vi "Import State.vi"(0 "SystemLink connection in":T1, 5 "state filepath":path, 7 "state name":string, 9 "state description":string, 11 "error in (no error)":errorcluster) -> (4 "SystemLink connection out":T1, 6 "state metadata":string, 15 "error out":errorcluster)   [LabVIEW 2017, in "SystemLink_States_API.lvlib"]
doc: "Imports the specified state file (.sls) on disk into the SystemLink server"
uses:
  SystemLink_States_API.lvlib
  _support/systemlink connection.ctl
  <vilib>/httpClient/ClientHandle.ctl
  <vilib>/httpClient/POSTBuffer.vi
  <vilib>/httpClient/LabVIEWHTTPClient.lvlib
panel:
  out "body":string
  out "headers":string
  # "The Import State VI does not work yet.  Need to better research how to implement the Import State HTTP API in LabVIEW\nImport State HTTP API: http://demo.systemlink.io/niapis/?urls.primaryName=Systems%20State%20Manager%20Service#/states/ImportState"
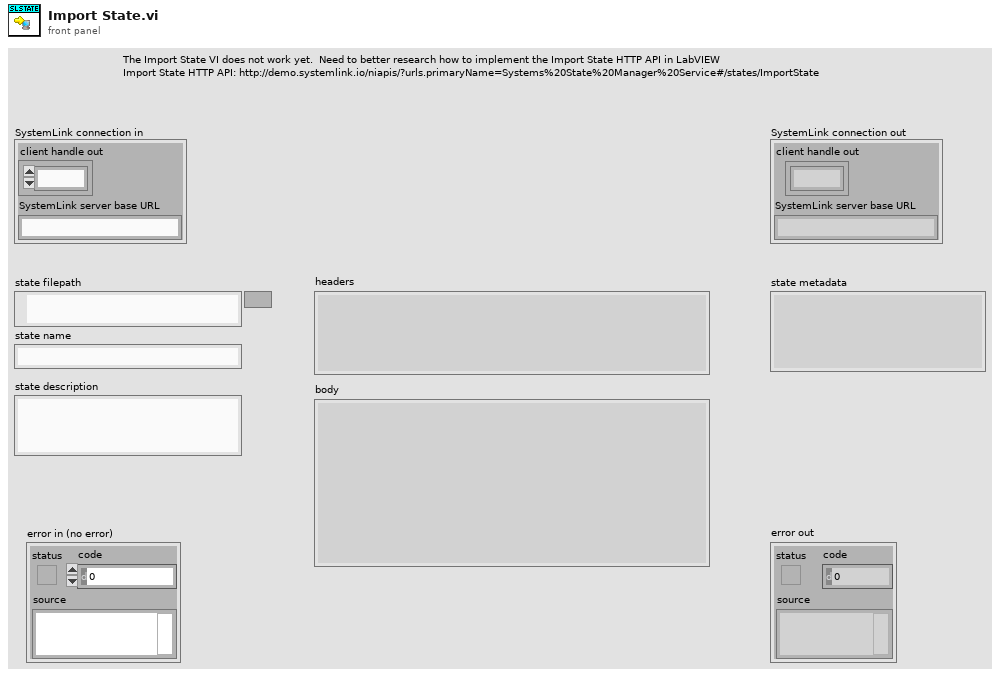
[diagram p1: front panel]
types:
  T1 = typedef "SystemLink_States_API.lvlib/systemlink connection.ctl" = cluster{"client handle out":T2, "SystemLink server base URL":string}
  T2 = typedef "LabVIEWHTTPClient.lvlib/ClientHandle.ctl" = refnum<k1>
  T3 = cluster{"file":string, "name":string, "description":string, "architecture":string}
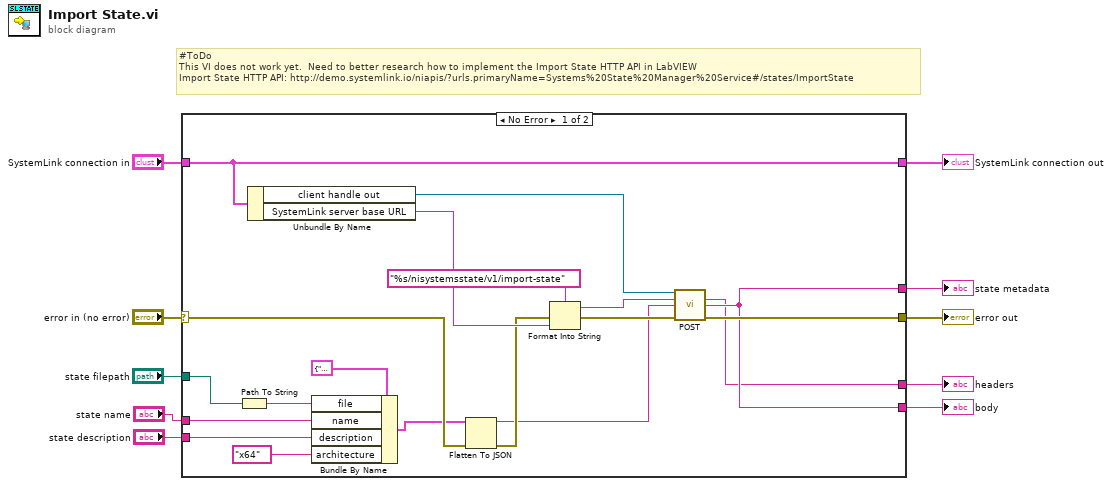
[diagram p0: block diagram]
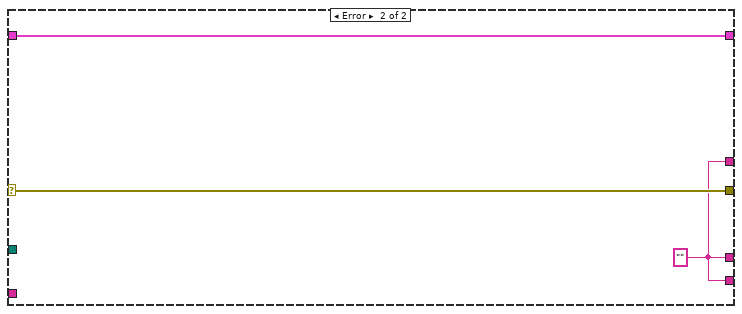
[diagram p2: hidden frame]
diagram:
  # "#ToDo\nThis VI does not work yet.  Need to better research how to implement the Import State HTTP API in LabVIEW\nImport State HTTP API: http://demo.systemlink.io/niapis/?urls.primaryName=Systems%20State%20Manager%20Service#/states/ImportState"
  n1 = case shown="No Error" "error in (no error)" {
    selector: "error in (no error)" -> [w19 w32]
    tunnel: "SystemLink connection in" -> [w21 w30]
    tunnel: [w25 w32] -> w9
    tunnel: [w23 w31] -> w5
    tunnel: [w23 w31] -> w8
    tunnel: [w22 w31] -> w7
    tunnel: "state filepath" -> [w16 _]
    tunnel: [w21 w30] -> w3
    tunnel: "state name" -> [w15 _]
    tunnel: "state description" -> [w13 _]
    frame No Error {
      n2 = Path To String(path=w16) -> (string=w11:string)
      n3 = Unbundle By Name(w21) -> ("client handle out"=w27:T2, "SystemLink server base URL"=w24:string)
      n4 = Bundle By Name(cluster=T3 {"file"="", "name"="", "description"="", "architecture"=""}, "file"=w11, "name"=w15, "description"=w13, "architecture"="x64" ("Combo Box")) -> (w12:T3)
      n5 = Flatten To JSON(anything=w12, error in (no error)=w19) -> (JSON string=w17:string, 11:w18:errorcluster)  [unwired: 1 in]
      n6 = Format Into String(format string="%s/nisystemsstate/v1/import-state", error in=w18, w24) -> (resulting string=w28:string, error out=w26:errorcluster)  [unwired: 1 in]
      n7 = call-poly <vilib>:"POST.vi"("client handle"=w27, "url"=w28, "buffer"=w17, "error in (no error)"=w26) -> ("headers"=w22:string, "body"=w23:string, "error out"=w25:errorcluster)  [unwired: 8 in, 1 out]
    }
    frame Error {
      w31 = "" ("headers")
    }
  }
  "error out" <- w9
  "SystemLink connection out" <- w3
  "headers" <- w7
  "body" <- w8
  "state metadata" <- w5
